vi "PID Modified.vi"(3 "reinitialize? (F)":bool, 4 "autotune? (F)":bool, 5 "output range":cluster{"output high":dbl, "output low":dbl}={"output high"=300.0, "output low"=0.0} {"output low" format="%.2f"; "output high" format="%.2f"}, 6 "PID Gains In":T1={"proportional gain (Kc)"=-1.0, "integral time (Ti, min)"=0.1, "derivative time (Td, min)"=0.0} {"derivative time (Td, min)" format="%.3f"; "integral time (Ti, min)" format="%.3f"; "proportional gain (Kc)" format="%.3f"}, 7 "Diff Press Setpoint":dbl=40.0 format="%.2f", 8 "Supply Pressure":dbl, 9 "Tolerance":dbl=0.1 format="%.3f", 10 "Differential Pressure":dbl) -> (0 "output":dbl, 1 "In Range?":bool=TRUE, 2 "PID gains out":T1={"proportional gain (Kc)"=1.0, "integral time (Ti, min)"=0.01, "derivative time (Td, min)"=0.0} {"derivative time (Td, min)" format="%.3f"; "integral time (Ti, min)" format="%.3f"; "proportional gain (Kc)" format="%.3f"})   [LabVIEW 2010]
uses:
  <vilib>/addons/control/pid/NI_PID_autopid.lvlib
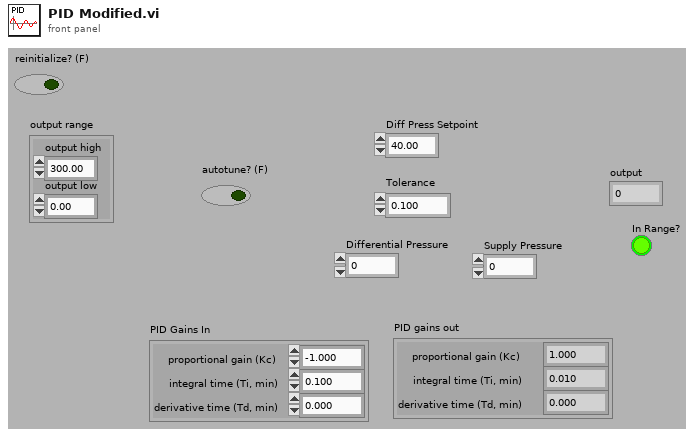
[diagram p1: front panel]
types:
  T1 = cluster{"proportional gain (Kc)":dbl, "integral time (Ti, min)":dbl, "derivative time (Td, min)":dbl}
  T2 = enum16{"get data", "set all data", "set Process Variable", "initialize"}
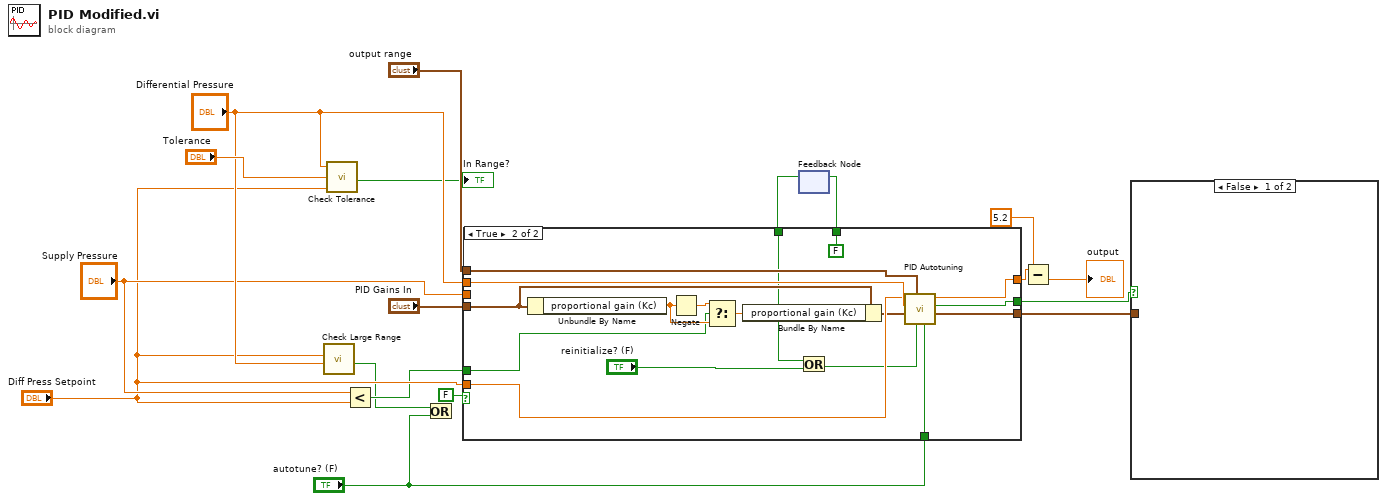
[diagram p0: block diagram]
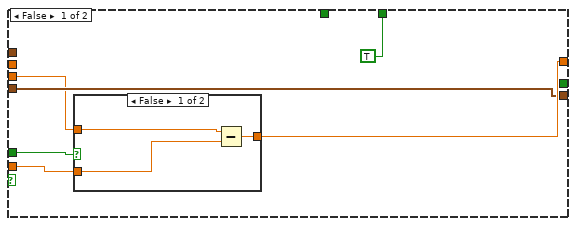
[diagram p2: hidden frame]
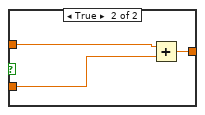
[diagram p3: hidden frame]
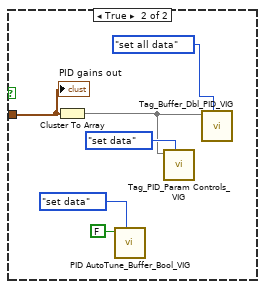
[diagram p4: hidden frame]
diagram:
  n1 = call "Check Large Range.vi"("Differential Pressure"="Differential Pressure", "Diff Press Setpoint"="Diff Press Setpoint") -> ("In Range?"=w4:bool)  [unwired: 9 in]
  n2 = call "Check Tolerance.vi"("setpoint"="Diff Press Setpoint", "Tolerance"="Tolerance", "Process variable"="Differential Pressure") -> ("Boolean"=→"In Range?":bool)
  n3 = Less?(x="Supply Pressure", y="Diff Press Setpoint") -> (x < y?=w7:bool)
  n4 = Or(x=w4, y="autotune? (F)") -> ()  [unwired: 1 out]
  n5 = feedback #1() -> (w5:bool)  [unwired: 1 in]
  n6 = case shown="True" FALSE {
    tunnel: "PID Gains In" -> [w23 w40]
    tunnel: "output range" -> [_ w47]
    tunnel: [w24 w46] -> w16
    tunnel: [w23 w44] -> w14
    tunnel: [_ w43] -> w13
    tunnel: "Differential Pressure" -> [_ w42]
    tunnel: "Diff Press Setpoint" -> [w22 w41]
    tunnel: w7 -> [w21 w35]
    tunnel: "Supply Pressure" -> [w20 _]
    tunnel: "autotune? (F)" -> [_ w34]
    tunnel: [TRUE FALSE] -> w6
    tunnel: w5 -> [_ w31]
    frame False {
      n7 = case shown="False" w21 {
        tunnel: [w27 w30] -> w24
        tunnel: w22 -> [w26 w29]
        tunnel: w20 -> [w25 w28]
        frame False {
          n8 = Subtract(x=w25, y=w26) -> (x-y=w27:dbl)
        }
        frame True {
          n9 = Add(x=w28, y=w29) -> (x+y=w30:dbl)
        }
      }
    }
    frame True {
      n10 = Unbundle By Name(w40) -> ("proportional gain (Kc)"=w38:dbl)
      n11 = Negate(x=w38) -> (-x=w39:dbl)
      n12 = Select(t=w39, s=w35, f=w38) -> (s? t:f=w36:dbl)
      n13 = Bundle By Name(cluster=w40, "proportional gain (Kc)"=w36) -> (w37:T1)
      n14 = Or(x=w31, y="reinitialize? (F)") -> (x .or. y?=w32:bool)
      n15 = call <vilib>:"PID Autotuning.vi"("autotune? (F)"=w34, "reinitialize? (F)"=w32, "output range"=w47, "PID gains"=w37, "process variable"=w42, "setpoint"=w41) -> ("PID gains out"=w44:T1, "tuning completed?"=w43:bool, "output"=w46:dbl)  [unwired: 2 in, 1 out]
    }
  }
  n16 = feedback-in #1(w6) -> ()
  n17 = Subtract(x=w16, y=5.2 ("x")) -> (x-y=→"output":dbl)
  n18 = case shown="False" w13 {
    tunnel: w14 -> [_ w53]
    frame False {
    }
    frame True {
      n19 = Cluster To Array(cluster=w53) -> (array=w50:dbl[])
      n20 = call "PID AutoTune_Buffer_Bool_VIG.vi"("Operation"=enum16{"get data", "set data", "initialize"}."set data", "Boolean"=FALSE) -> ()  [unwired: 8 in, 2 out]
      n21 = call "Tag_PID_Param Controls_VIG.vi"("Operation"=enum16{"get data", "set data", "initialize"}."set data", "tag_data_in"=w50) -> ()  [unwired: 8 in, 2 out]
      n22 = call "Tag_Buffer_Dbl_PID_VIG.vi"("Operation"=T2."set all data", "tag_data_in"=w50) -> ()  [unwired: 8 in, 2 out]
      "PID gains out" <- w53
    }
  }
